vi "Boolean To String.vi"(11 "1D Boolean Array":bool[](array[boolean])) -> (3 "Binary String":string)   [LabVIEW 2021]
doc: "Converts a 1D string of booleans into a string."
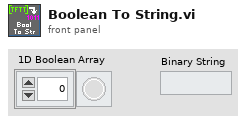
[diagram p1: front panel]
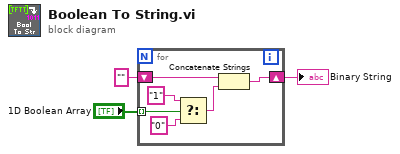
[diagram p0: block diagram]
diagram:
  n1 = for {
    tunnel: "1D Boolean Array" -> [w9] mode=indexing
    shift-right: [w5] -> w1
    shift-left: "" -> [w4]
    n2 = Select(t="1", s=w9, f="0") -> (s? t:f=w6:string)
    n3 = Concatenate Strings(w4, w6) -> (w5:string)
  }
  "Binary String" <- w1
